vi "Circle detect Auto Flight (SubVI).vi"(10 "element":T1, 11 "Number of Matches Returned":i32) -> (3 "Control Cluster out":T2 {"Yaw Speed" scale=-1.0..1.0; "Vertical Speed" scale=-1.0..1.0; "Pitch" scale=-1.0..1.0; "Roll" scale=-1.0..1.0})   [LabVIEW 2014]
uses:
  Others/Control cluster.ctl
  Global.vi
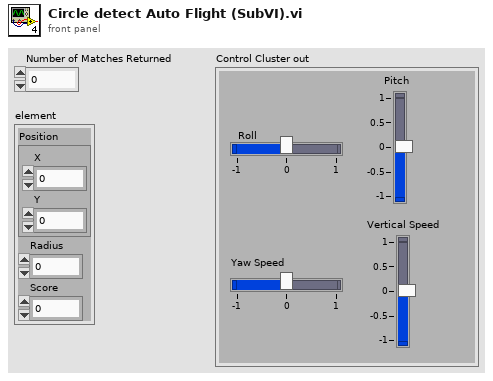
[diagram p1: front panel]
types:
  T1 = cluster{"Position":cluster{"X":sgl, "Y":sgl}, "Radius":dbl, "Score":dbl}
  T2 = typedef "Control cluster.ctl" = cluster{"Roll":sgl, "Pitch":sgl, "Vertical Speed":sgl, "Yaw Speed":sgl}
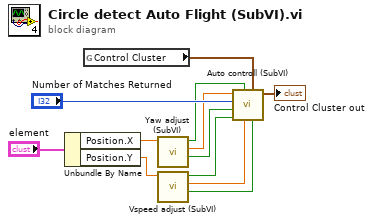
[diagram p0: block diagram]
diagram:
  n1 = Unbundle By Name("element") -> ("Position.X"=w5:sgl, "Position.Y"=w4:sgl)
  n2 = global read "Global.vi" "Control Cluster"() -> (w10:T2)
  n3 = call "Yaw adjust (SubVI).vi"("X"=w5) -> ("Boolean"=w8:bool, "Numeric"=w7:dbl, "Boolean 2"=w6:bool)  [unwired: 8 in]
  n4 = call "Vspeed adjust (SubVI).vi"("Y"=w4) -> ("Boolean"=w12:bool, "Numeric"=w11:dbl, "Boolean 2"=w3:bool)  [unwired: 8 in]
  n5 = call "Auto controll (SubVI).vi"("Boolean"=w12, "Control Cluster in"=w10, "Numeric"=w11, "Boolean 3"=w6, "Boolean 4"=w3, "Boolean 2"=w8, "Number of Matches Returned"="Number of Matches Returned", "Numeric 2"=w7) -> ("Control Cluster out"=→"Control Cluster out":T2)  [unwired: 3 in]
